vi "Enable or Disable.vi"(0 "Condition":bool) -> (4 "Disabled":T1(ring))   [LabVIEW 2018, in "Embedded Data Logger System Explorer.lvlib"]
uses:
  Embedded Data Logger System Explorer.lvlib
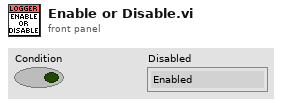
[diagram p1: front panel]
types:
  T1 = enum8{"Enabled", "Disabled", "Disabled and Grayed Out"}
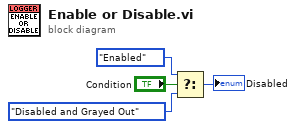
[diagram p0: block diagram]
diagram:
  n1 = Select(t=T1."Enabled" ("Disabled"), s="Condition", f=T1."Disabled and Grayed Out" ("Disabled")) -> (s? t:f=→"Disabled":T1)
